vi "Test Acquisition API.vi"() -> ()   [LabVIEW 2019]
doc: "Acquisition API Tester.\n_____\nBased on Delacor QMH Project Template 5.0.0.82."
uses:
  Acquisition.lvlib
  Settings Editor/Settings Editor.lvlib
panel:
  in  "Settings":bool
  out "error out":errorcluster
  out "Calibrated?":bool
  in  "Calibrate":bool
  out "Waveform Chart":waveform(dbl)[](graph)
  out "Acquiring?":bool
  in  "Stop Acquiring":bool
  out "HW ID":string
  in  "Start Acquiring":bool
  in  "Show Block Diagram":bool
  in  "Stop Module":bool
  in  "Start Module":bool
  in  "Hide Module Panel":bool
  in  "Show Module Panel":bool
  out "Status":string
  out "Module Running?":bool
  # "This VI tests the API for the Module."
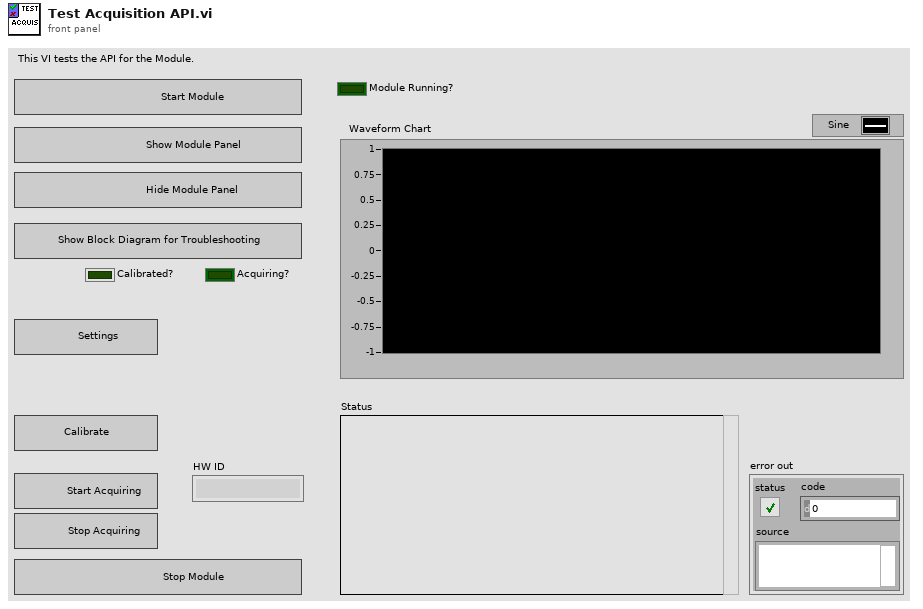
[diagram p1: front panel]
types:
  T1 = typedef "Acquisition.lvlib/Broadcast Events--cluster.ctl" = cluster{"Module Did Init":refnum<user-event>, "Status Updated":refnum<user-event>, "Error Reported":refnum<user-event>, "Module Did Stop":refnum<user-event>, "Update Module Execution Status":refnum<user-event>, "Acquisition Started":refnum<user-event>, "Acquisition Stopped":refnum<user-event>, "Data Updated":refnum<user-event>, "Device Calibrated":refnum<user-event>}
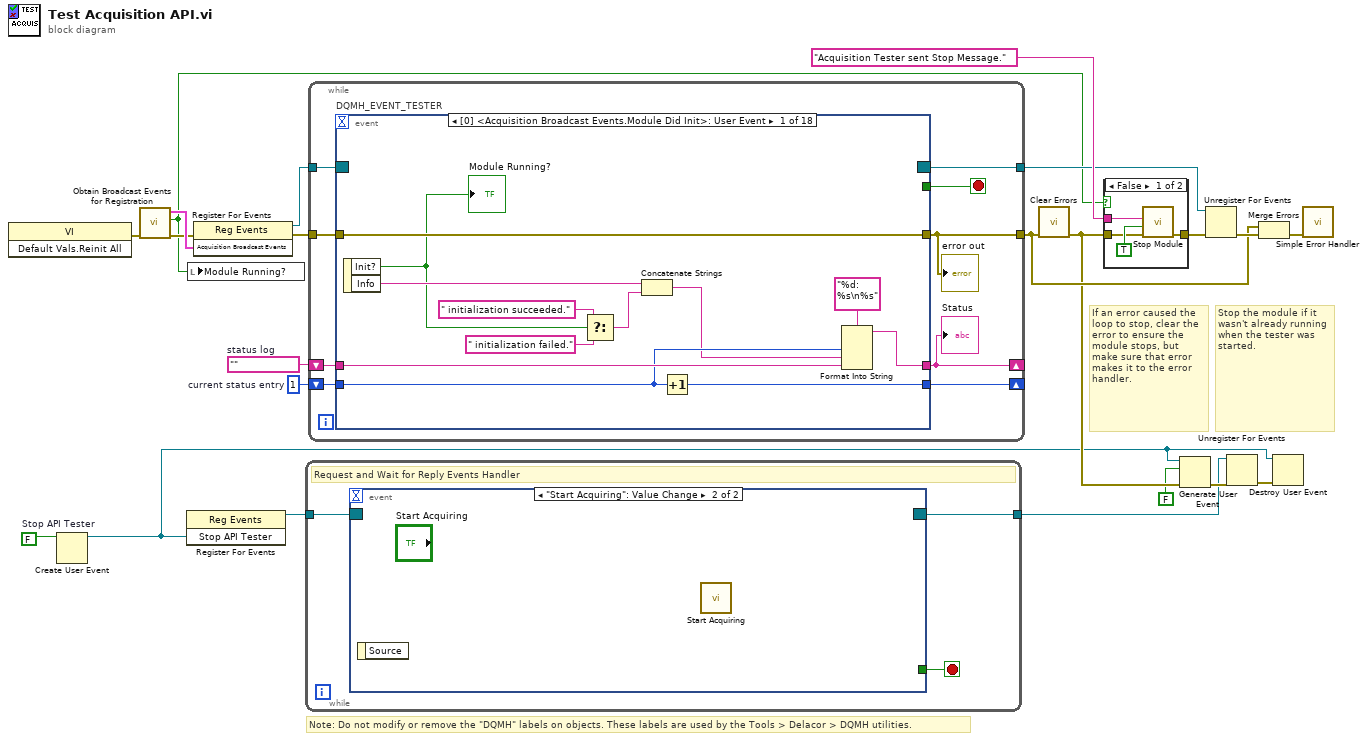
[diagram p0: block diagram]
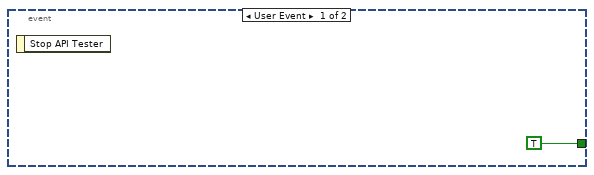
[diagram p3: hidden frame]
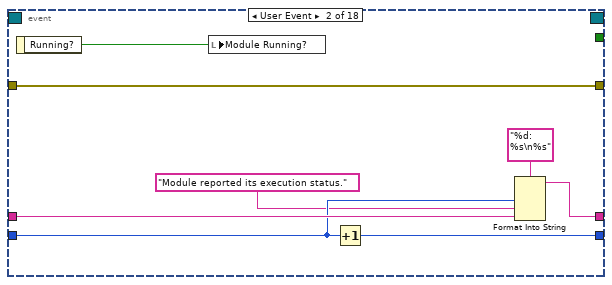
[diagram p4: hidden frame]
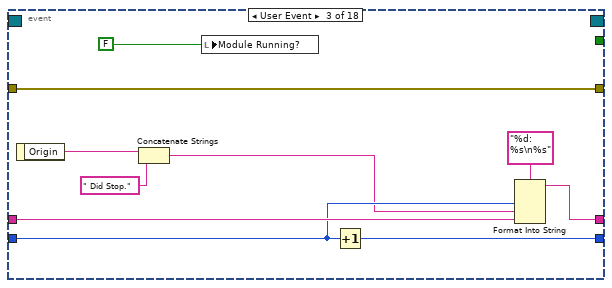
[diagram p5: hidden frame]
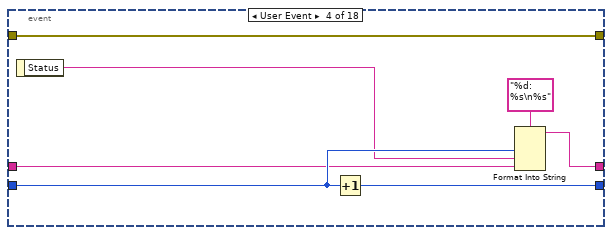
[diagram p6: hidden frame]
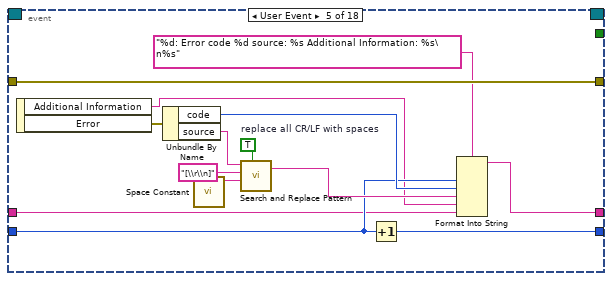
[diagram p7: hidden frame]
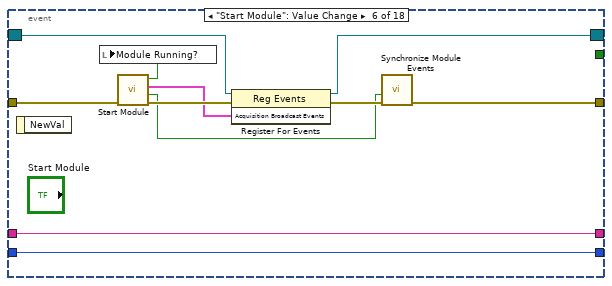
[diagram p8: hidden frame]
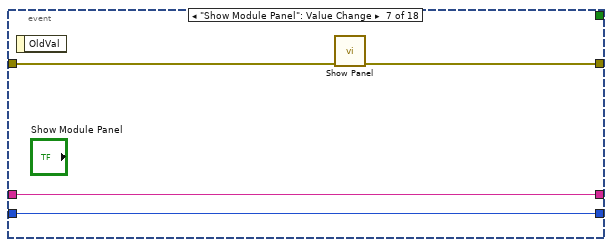
[diagram p9: hidden frame]
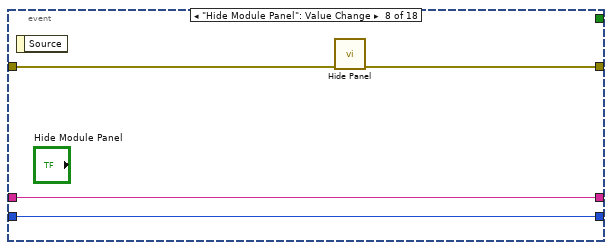
[diagram p10: hidden frame]
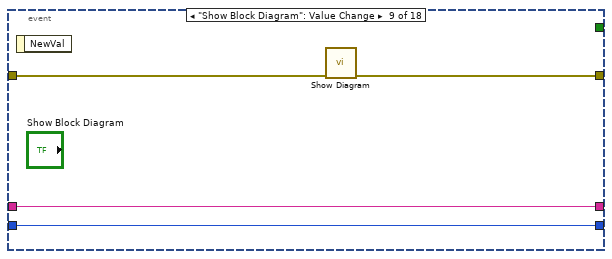
[diagram p11: hidden frame]
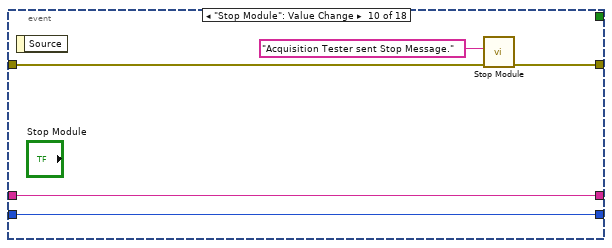
[diagram p12: hidden frame]
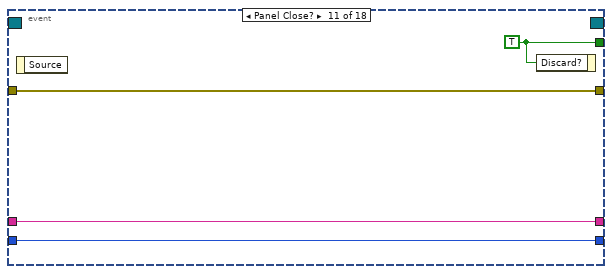
[diagram p13: hidden frame]
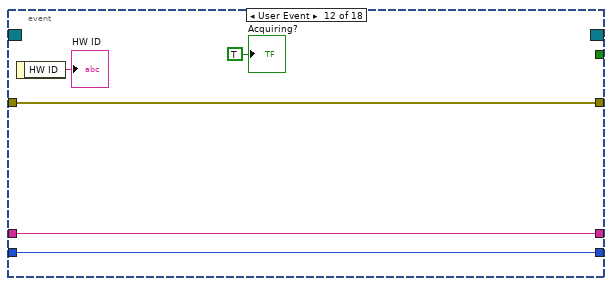
[diagram p14: hidden frame]
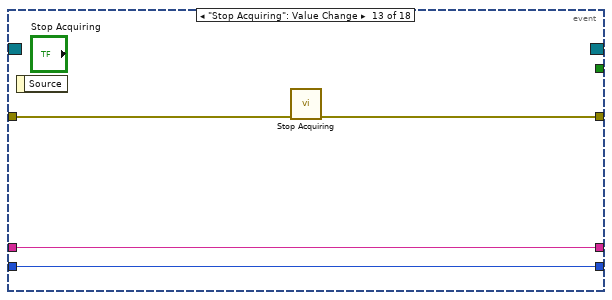
[diagram p15: hidden frame]
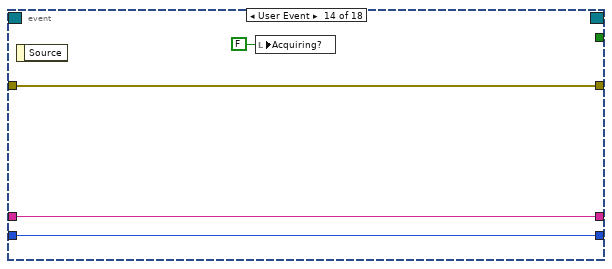
[diagram p16: hidden frame]
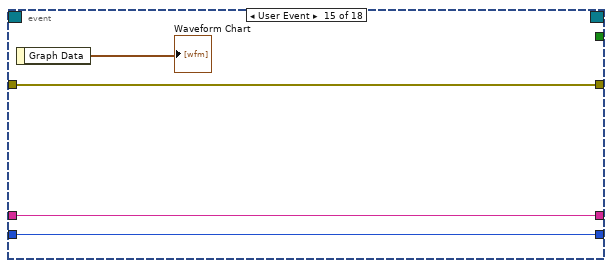
[diagram p17: hidden frame]
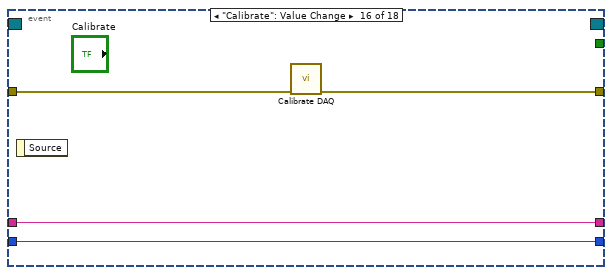
[diagram p18: hidden frame]
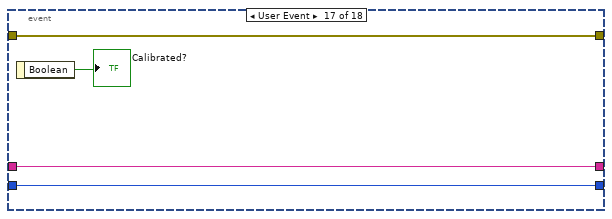
[diagram p19: hidden frame]
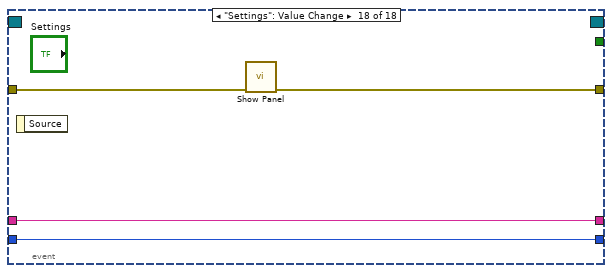
[diagram p20: hidden frame]
diagram:
  w9 = FALSE  # Stop API Tester
  w18 = 1  # current status entry
  w19 = ""  # status log
  # "Stop the module if it wasn't already running when the tester was started."
  # "If an error caused the loop to stop, clear the error to ensure the module stops, but make sure that error makes it to the error handler."
  # "Note: Do not modify or remove the \"DQMH\" labels on objects. These labels are used by the Tools > Delacor > DQMH utilities."
  n1 = invoke on="Invoke Node" class="VI" method="Default Vals.Reinit All"() -> (error out=w11:errorcluster)  [unwired: 3 in, 2 out]
  n2 = Create User Event(user event datatype=w9) -> (user event=w2:refnum<user-event>)  [unwired: 1 in, 1 out]
  n3 = call "Obtain Broadcast Events for Registration.vi"("error in (no error)"=w11) -> ("error out"=w10:errorcluster, "Already running?"=w1:bool, "Acquisition Broadcast Events"=w16:T1)  [unwired: 8 in]
  n4 = register-events(w2) -> (reference out=w8:refnum<event-registration>)  [unwired: 2 in, 1 out]
  n5 = local write "Module Running?"(w1) -> ()
  n6 = register-events(error in=w10, w16) -> (reference out=w15:refnum<event-registration>, error out=w17:errorcluster)  [unwired: 1 in]
  n7 = while {
    tunnel: w8 -> [w25]
    tunnel: [w23] -> w4
    stop <- w24 stop-if-true
    # "Request and Wait for Reply Events Handler"
    n8 = event shown="[1] \"Start Acquiring\": Value Change" {
      selector: w25 -> [_ _]
      dyn-events: [_ _] -> w23
      timeout: _ -> [_ _]
      tunnel: [TRUE _] -> w24
      event User Event {
        n9 = event-data() -> ()  [unwired: 1 in, 1 out]
      }
      event "Start Acquiring": Value Change {
        n10 = event-data() -> ()  [unwired: 1 in, 1 out]
        n11 = call "Start Acquiring.vi"() -> ()  [unwired: 9 in, 3 out]
      }
    }
  }
  n12 = while {
    tunnel: w15 -> [w35]
    tunnel: [w28] -> w12
    shift-right: [w31] -> _
    shift-left: w19 -> [w33]
    shift-right: [w32] -> _
    shift-left: w18 -> [w34]
    tunnel: w17 -> [w30]
    tunnel: [w29] -> w14
    stop <- w27 stop-if-true
    n13 = event "DQMH_EVENT_TESTER" shown="[0] <Acquisition Broadcast Events.Module Did Init>: User Event" {
      selector: w35 -> [_ _ _ _ _ w91 _ _ _ _ _ _ _ _ _ _ _ _]
      dyn-events: [_ _ _ _ _ w90 _ _ _ _ _ _ _ _ _ _ _ _] -> w29
      timeout: _ -> [_ _ _ _ _ _ _ _ _ _ _ _ _ _ _ _ _ _]
      tunnel: [_ _ _ _ _ _ _ _ _ _ w118 _ _ _ _ _ _ _] -> w27
      tunnel: [w47 w49 w56 w66 w86 w89 w101 w105 w106 w112 w115 w123 w124 w131 w135 w136 w143 w144] -> w28
      tunnel: w34 -> [w44 w53 w63 w69 w76 w94 w99 w103 w107 w113 w116 w121 w125 w129 w133 w137 w141 w146]
      tunnel: w33 -> [w45 w54 w64 w68 w74 w95 w100 w104 w108 w114 w117 w122 w126 w130 w134 w138 w142 w147]
      tunnel: [w42 w51 w61 w70 w77 w95 w100 w104 w108 w114 w117 w122 w126 w130 w134 w138 w142 w147] -> w31
      tunnel: [w43 w52 w62 w72 w75 w94 w99 w103 w107 w113 w116 w121 w125 w129 w133 w137 w141 w146] -> w32
      tunnel: w30 -> [w47 w49 w56 w66 w86 w88 w98 w102 w109 w110 w115 w123 w127 w131 w135 w139 w143 w145]
      event User Event {
        n14 = event-data() -> ("Init?"=w39:bool, "Info"=w41:string)  [unwired: 1 in]
        "Module Running?" <- w39
        n15 = Select(t=" initialization succeeded.", s=w39, f=" initialization failed.") -> (s? t:f=w36:string)
        n16 = Concatenate Strings(w41, w36) -> (w40:string)
        n17 = Increment(x=w44) -> (x+1=w43:i32)
        n18 = Format Into String(format string="%d: %s\n%s", w44, w40, w45) -> (resulting string=w42:string)  [unwired: 2 in, 1 out]
      }
      event User Event {
        n19 = event-data() -> ("Running?"=w48:bool)  [unwired: 1 in]
        n20 = local write "Module Running?"(w48) -> ()
        n21 = Increment(x=w53) -> (x+1=w52:i32)
        n22 = Format Into String(format string="%d: %s\n%s", w53, "Module reported its execution status.", w54) -> (resulting string=w51:string)  [unwired: 2 in, 1 out]
      }
      event User Event {
        n23 = event-data() -> ("Origin"=w60:string)  [unwired: 1 in]
        n24 = Concatenate Strings(w60, " Did Stop.") -> (w59:string)
        n25 = local write "Module Running?"(FALSE ("Module Did Init?")) -> ()
        n26 = Increment(x=w63) -> (x+1=w62:i32)
        n27 = Format Into String(format string="%d: %s\n%s", w63, w59, w64) -> (resulting string=w61:string)  [unwired: 2 in, 1 out]
      }
      event User Event {
        n28 = event-data() -> ("Status"=w67:string)  [unwired: 1 in]
        n29 = Increment(x=w69) -> (x+1=w72:i32)
        n30 = Format Into String(format string="%d: %s\n%s", w69, w67, w68) -> (resulting string=w70:string)  [unwired: 2 in, 1 out]
      }
      event User Event {
        w82 = TRUE  # replace all CR/LF with spaces
        n31 = event-data() -> ("Additional Information"=w73:string, "Error"=w78:errorcluster)  [unwired: 1 in]
        n32 = Unbundle By Name(w78) -> ("code"=w79:i32, "source"=w80:string)
        n33 = call <vilib>:"Space Constant.vi"() -> ("String"=w83:string)
        n34 = call <vilib>:"Search and Replace Pattern.vi"("string"=w80, "regular expression (\"\")"="[\\r\\n]" ("regular expression (\"\")"), "replace string (\"\")"=w83, "replace all? (F)"=w82) -> ("result string"=w81:string)  [unwired: 1 in, 1 out]
        n35 = Increment(x=w76) -> (x+1=w75:i32)
        n36 = Format Into String(format string="%d: Error code %d source: %s Additional Information: %s\n%s", w76, w79, w81, w73, w74) -> (resulting string=w77:string)  [unwired: 2 in, 1 out]
      }
      event "Start Module": Value Change {
        n37 = event-data() -> ()  [unwired: 1 in, 1 out]
        n38 = call "Start Module.vi"("error in (no error)"=w88) -> ("error out"=w96:errorcluster, "Wait for Event Sync?"=w93:bool, "Acquisition Broadcast Events"=w92:T1, "Module Was Already Running?"=w87:bool)  [unwired: 7 in]
        n39 = local write "Module Running?"(w87) -> ()
        n40 = register-events(reference=w91, error in=w96, w92) -> (reference out=w90:refnum<event-registration>, error out=w97:errorcluster)
        n41 = call "Synchronize Module Events.vi"("error in (no error)"=w97, "Wait for Event Sync?"=w93) -> ("error out"=w89:errorcluster)  [unwired: 9 in]
      }
      event "Show Module Panel": Value Change {
        n42 = event-data() -> ()  [unwired: 1 in, 1 out]
        n43 = call "Show Panel.vi"("error in (no error)"=w98) -> ("error out"=w101:errorcluster)  [unwired: 10 in]
      }
      event "Hide Module Panel": Value Change {
        n44 = event-data() -> ()  [unwired: 1 in, 1 out]
        n45 = call "Hide Panel.vi"("error in (no error)"=w102) -> ("error out"=w105:errorcluster)  [unwired: 10 in]
      }
      event "Show Block Diagram": Value Change {
        n46 = event-data() -> ()  [unwired: 1 in, 1 out]
        n47 = call "Show Diagram.vi"("error in (no error)"=w109) -> ("error out"=w106:errorcluster)  [unwired: 10 in]
      }
      event "Stop Module": Value Change {
        n48 = event-data() -> ()  [unwired: 1 in, 1 out]
        n49 = call "Stop Module.vi"("error in (no error)"=w110, "Origin"="Acquisition Tester sent Stop Message.") -> ("error out"=w112:errorcluster)  [unwired: 9 in]
      }
      event Panel Close? {
        w118 = TRUE ("Discard?")
        n50 = event-data() -> ()  [unwired: 1 in, 1 out]
        n51 = event-data ("Event Filter Node")("Discard?"=w118) -> ()  [unwired: 1 in, 1 out]
      }
      event User Event {
        n52 = event-data() -> ("HW ID"=→"HW ID":string)  [unwired: 1 in]
        "Acquiring?" <- TRUE ("Acquiring?")
      }
      event "Stop Acquiring": Value Change {
        n53 = event-data() -> ()  [unwired: 1 in, 1 out]
        n54 = call "Stop Acquiring.vi"("error in (no error)"=w127) -> ("error out"=w124:errorcluster)  [unwired: 10 in]
      }
      event User Event {
        n55 = event-data() -> ()  [unwired: 1 in, 1 out]
        n56 = local write "Acquiring?"(FALSE ("Acquiring?")) -> ()
      }
      event User Event {
        n57 = event-data() -> ("Graph Data"=→"Waveform Chart":waveform(dbl)[])  [unwired: 1 in]
      }
      event "Calibrate": Value Change {
        n58 = event-data() -> ()  [unwired: 1 in, 1 out]
        n59 = call "Calibrate DAQ.vi"("error in (no error)"=w139) -> ("error out"=w136:errorcluster)  [unwired: 10 in]
      }
      event User Event {
        n60 = event-data() -> ("Boolean"=→"Calibrated?":bool)  [unwired: 1 in]
      }
      event "Settings": Value Change {
        n61 = event-data() -> ()  [unwired: 1 in, 1 out]
        n62 = call "Show Panel.vi"("error in (no error)"=w145) -> ("error out"=w144:errorcluster)  [unwired: 10 in]
      }
    }
    "Status" <- w31
    "error out" <- w28
  }
  n63 = call <vilib>:"Clear Errors.vi"("error in (no error)"=w12) -> ("error out"=w7:errorcluster)  [unwired: 5 in, 1 out]
  n64 = case shown="False" w1 {
    tunnel: [w151 w152] -> w21
    tunnel: "Acquisition Tester sent Stop Message." ("Origin") -> [w150 _]
    tunnel: w7 -> [w148 w152]
    frame False {
      n65 = call "Stop Module.vi"("error in (no error)"=w148, "Wait for Module to Stop? (F)"=TRUE ("Wait for Module to stop?"), "Origin"=w150) -> ("error out"=w151:errorcluster)  [unwired: 8 in]
    }
    frame True {
    }
  }
  n66 = Generate User Event(user event=w2, event data cluster=FALSE ("Stop API Tester"), error in=w7) -> (error out=w5:errorcluster)  [unwired: 1 in, 1 out]
  n67 = Unregister For Events(event registration refnum=w14, error in=w21) -> (error out=w22:errorcluster)
  n68 = Unregister For Events(event registration refnum=w4, error in=w5) -> (error out=w3:errorcluster)
  n69 = Merge Errors(w12, w22) -> (w13:errorcluster)
  n70 = Destroy User Event(user event=w2, error in=w3) -> ()  [unwired: 1 out]
  n71 = call <vilib>:"Simple Error Handler.vi"("error in (no error)"=w13) -> ()  [unwired: 4 in, 5 out]
